vi "Actor Core.vi"(8 "error in":errorcluster, 11 "ePAS in":refnum<class "ePAS.lvclass">) -> (0 "error out":errorcluster, 3 "Actor out":refnum<class "Actor.lvclass">)   [LabVIEW 2014, in "PAS Actor Lib.lvlib" / "ePAS.lvclass"]
doc: "(<B>Filename</B>: Actor Framework.lvlib:Actor.lvclass:Actor Core.vi)\n\nReceives messages to the actor, reacts to them, and initiates any error handling that may shut the actor down.\n\nDescendant classes may override this VI to append parallel tasks for the actor to complete while it handles messages. Overrides use the Call Parent Method node."
uses:
  ePAS.lvclass
  reusable/Instrument/Instrument.lvclass
  reusable/PAS/Main/PAS.lvclass
  reusable/Instrument/state.ctl
  <vilib>/ActorFramework/Actor/Actor.lvclass
  Messages/Data MSG/Data MSG.lvclass
  <vilib>/ActorFramework/Message Enqueuer/Message Enqueuer.lvclass
  Instr Actor/Instr Actor.lvclass
  reusable/Command/Command.lvclass
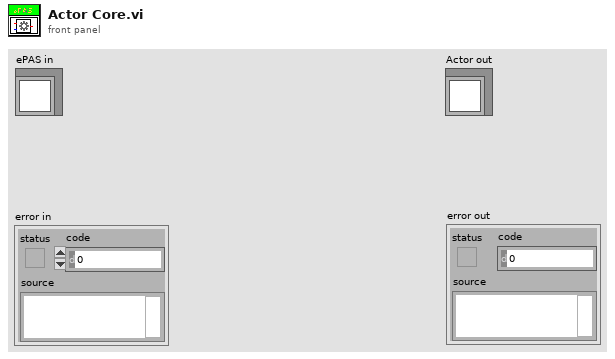
[diagram p1: front panel]
types:
  T1 = typedef "Instrument.lvclass/state.ctl" = enum8{"Configure", "Acquire", "Wait", "Quit", "Handle Error", "NOOP"}
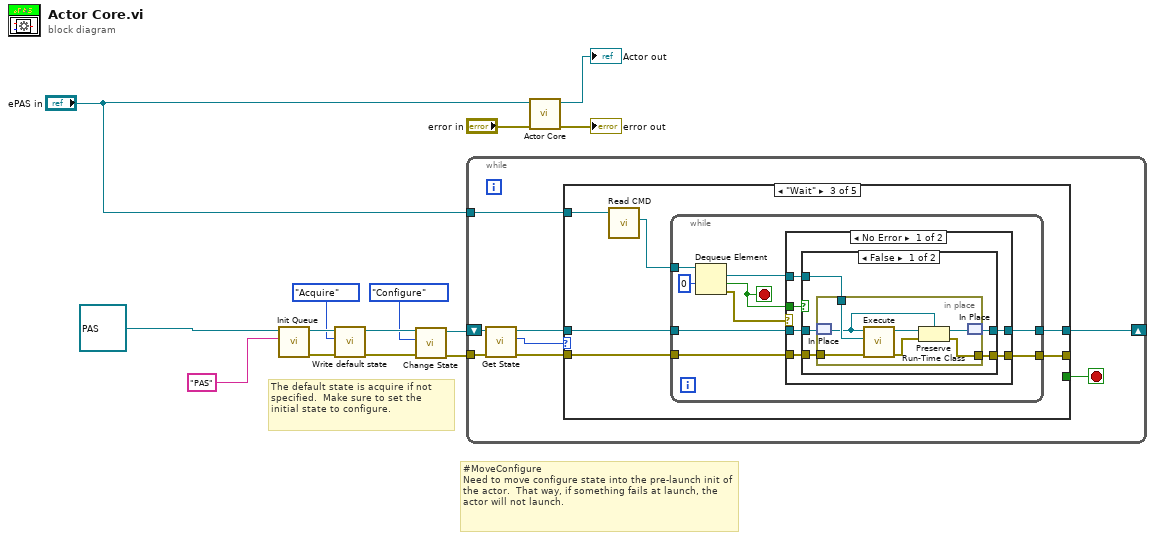
[diagram p0: block diagram]
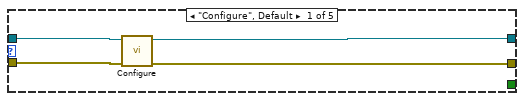
[diagram p2: hidden frame]
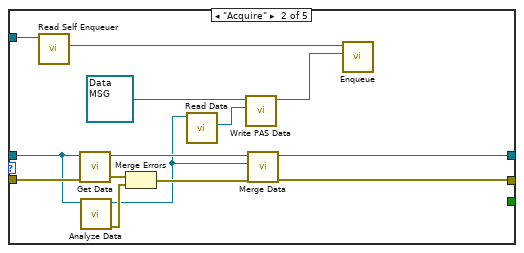
[diagram p3: hidden frame]
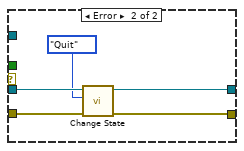
[diagram p5: hidden frame]
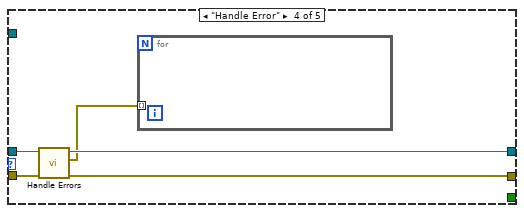
[diagram p6: hidden frame]
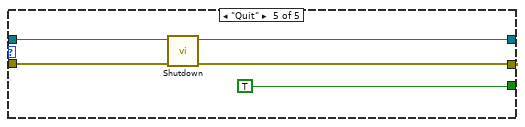
[diagram p7: hidden frame]
diagram:
  # "#MoveConfigure\nNeed to move configure state into the pre-launch init of the actor.  That way, if something fails at launch, the actor will not launch."
  # "The default state is acquire if not specified.  Make sure to set the initial state to configure."
  n1 = call "Init Queue.vi"("queue_name"="PAS", "Instrument in"=refnum<class "PAS.lvclass"> refnum ("PAS")) -> ("error out"=w8:errorcluster, "Instrument out"=w9:refnum<class "Instrument.lvclass">)  [unwired: 8 in]
  n2 = call "Write default state.vi"("error in (no error)"=w8, "instr state"=state."Acquire", "Instrument in"=w9) -> ("error out"=w5:errorcluster, "Instrument out"=w6:refnum<class "Instrument.lvclass">)  [unwired: 7 in]
  n3 = call "Change State.vi"("error in"=w5, "instr state"=state."Configure", "Instrument in"=w6) -> ("error out"=w3:errorcluster, "Instrument out"=w4:refnum<class "Instrument.lvclass">)  [unwired: 7 in]
  n4 = while "Acquisition" {
    tunnel: w3 -> [w22]
    shift-right: [w16] -> _
    shift-left: w4 -> [w20]
    tunnel: "ePAS in" -> [w15]
    stop <- w17 stop-if-true
    n5 = call "Get State.vi"("error in"=w22, "Instrument in"=w20) -> ("error out"=w18:errorcluster, "default state"=w21:T1, "Instrument out"=w19:refnum<class "Instrument.lvclass">)  [unwired: 7 in]
    n6 = case shown="\"Wait\"" w21 {
      tunnel: w19 -> [w26 w39 w46 w85 w89]
      tunnel: w18 -> [w25 w40 w43 w84 w88]
      tunnel: [_ _ _ _ TRUE] -> w17
      tunnel: [w24 w35 w45 w82 w87] -> w16
      tunnel: [w23 w33 w44 w83 w86] -> _
      tunnel: w15 -> [_ w32 w42 _ _]
      frame "Configure", Default {
        n7 = call-dynamic "Configure.vi"("error in"=w25, "Instrument in"=w26) -> ("error out"=w23:errorcluster, "Instrument out"=w24:refnum<class "Instrument.lvclass">)  [unwired: 8 in]
      }
      frame "Acquire" {
        n8 = call <vilib>:"Read Self Enqueuer.vi"("Actor"=w32) -> ("Self Enqueuer"=w28:refnum<class "Message Enqueuer.lvclass">)  [unwired: 10 in]
        n9 = call-dynamic "Get Data.vi"("error in"=w40, "Instrument in"=w39) -> ("error out"=w38:errorcluster, "Instrument out"=w36:refnum<class "Instrument.lvclass">)  [unwired: 8 in]
        n10 = call-dynamic "Analyze Data.vi"("Instrument in"=w39) -> ("error out"=w37:errorcluster, "Instrument out"=w30:refnum<class "Instrument.lvclass">)  [unwired: 9 in]
        n11 = Merge Errors(w38, w37) -> (w34:errorcluster)
        n12 = call "Read Data.vi"("PAS in"=w30) -> ("PAS Data"=w29:refnum<class "PAS Data.lvclass">)  [unwired: 8 in, 2 out]
        n13 = call "Write PAS Data.vi"("DataIn"=w29, "Data MSG in"=refnum<class "Data MSG.lvclass"> refnum ("PAS Actor Lib.lvlib:Data MSG")) -> ("Data MSG out"=w27:refnum<class "Data MSG.lvclass">)  [unwired: 8 in, 1 out]
        n14 = call-dynamic "Merge Data.vi"("error in"=w34, "Analyzed"=w30, "Acquired"=w36) -> ("error out"=w33:errorcluster, "Instrument out"=w35:refnum<class "Instrument.lvclass">)  [unwired: 7 in]
        n15 = call <vilib>:"Enqueue.vi"("Message"=w27, "Message Enqueuer in"=w28) -> ()  [unwired: 8 in, 2 out]
      }
      frame "Wait" {
        n16 = call "Read CMD.vi"("Instr Actor in"=w42) -> ("CMD"=w41:refnum<queue>)  [unwired: 8 in, 2 out]
        n17 = while {
          tunnel: w41 -> [w55]
          tunnel: w46 -> [w54]
          tunnel: [w53] -> w45
          tunnel: [w51] -> w44
          tunnel: w43 -> [w50]
          stop <- w49 stop-if-true
          n18 = Dequeue Element(queue=w55, timeout in ms (-1)=0) -> (element=w52:refnum<class "Command.lvclass">, timed out?=w49:bool, error out=w48:errorcluster)  [unwired: 1 in, 1 out]
          n19 = case shown="No Error" w48 {
            tunnel: w54 -> [w61 w80]
            tunnel: [w60 w79] -> w53
            tunnel: w52 -> [w59 _]
            tunnel: [w58 w78] -> w51
            tunnel: w50 -> [w57 w77]
            tunnel: w49 -> [w56 _]
            frame No Error {
              n20 = case shown="False" w56 {
                tunnel: w61 -> [w66 w74]
                tunnel: [w65 w74] -> w60
                tunnel: w59 -> [w64 _]
                tunnel: [w63 w75] -> w58
                tunnel: w57 -> [w62 w75]
                frame False {
                  n21 = in-place {
                    in-place-border: w64 -> [w73]
                    in-place-border: [w68] -> w63
                    in-place-border: w62 -> [w67]
                    n22 = in-place-match #1(w66) -> (w72:refnum<class "Instrument.lvclass">)
                    n23 = call "Execute.vi"("error in"=w67, "Command in"=w73, "Object In"=w72) -> ("error out"=w69:errorcluster, "Object Out"=w71:refnum<class>)  [unwired: 7 in]
                    n24 = Preserve Run-Time Class(object in=w71, error in=w69, 2:w72) -> (object out=w70:refnum<class "Instrument.lvclass">, error out=w68:errorcluster)
                    n25 = in-place-match #1(w70) -> (w65:refnum<class "Instrument.lvclass">)
                  }
                }
                frame True {
                }
              }
            }
            frame Error {
              n26 = call "Change State.vi"("error in"=w77, "instr state"=state."Quit", "Instrument in"=w80) -> ("error out"=w78:errorcluster, "Instrument out"=w79:refnum<class "Instrument.lvclass">)  [unwired: 7 in]
            }
          }
        }
      }
      frame "Handle Error" {
        n27 = call-dynamic "Handle Errors.vi"("error in"=w84, "Instrument in"=w85) -> ("error out"=w83:errorcluster, "errors"=w81:errorcluster[], "Instrument out"=w82:refnum<class "Instrument.lvclass">)  [unwired: 7 in]
        n28 = for {
          tunnel: w81 -> [_] mode=indexing
        }
      }
      frame "Quit" {
        n29 = call-dynamic "Shutdown.vi"("error in"=w88, "Instrument in"=w89) -> ("error out"=w86:errorcluster, "Instrument out"=w87:refnum<class "Instrument.lvclass">)  [unwired: 8 in]
      }
    }
  }
  n30 = call-parent "Actor Core.vi"("error in"="error in", "Instr Actor in"="ePAS in") -> ("error out"=→"error out":errorcluster, "Actor out"=→"Actor out":refnum<class "Actor.lvclass">)  [unwired: 8 in]
